vi "I(V) at various fields_K6221-K2182A_PK.vi"() -> ()   [LabVIEW 2016]
uses:
  Labview Drivers/Keithley 622x LV 2009/Keithley 622x.lvlib
panel:
  in  "Numeric Average":i32=1
  out "Iset (A)":dbl=0.000246
  out "data":dbl[](array[numeric])=[-0.004996105, 0.000246, 1.09736792e-07, 0.0004460845203252032]
  out "I vs V":cluster{dbl, "Field Reading":dbl}[](graph)=[{0.0, "Field Reading"=4.05379385e-08}, {2e-06, "Field Reading"=3.64587619e-08}, {4e-06, "Field Reading"=2.9732457e-08}, {6e-06, "Field Reading"=3.98881058e-08}, {8e-06, "Field Reading"=2.30033844e-08}, {1e-05, "Field Reading"=4.97153356e-08}, {1.2e-05, "Field Reading"=4.75621284e-08}, {1.4e-05, "Field Reading"=5.84210222e-08}, {1.6e-05, "Field Reading"=2.26147627e-08}, {1.8e-05, "Field Reading"=5.23454209e-08}, {2e-05, "Field Reading"=6.56079851e-08}, {2.2e-05, "Field Reading"=2.92396798e-08}, {2.4e-05, "Field Reading"=4.16692625e-08}, {2.6e-05, "Field Reading"=4.41799263e-08}, {2.8e-05, "Field Reading"=7.01712601e-08}, {3e-05, "Field Reading"=6.50284783e-08}, {3.2e-05, "Field Reading"=5.58979313e-08}, {3.4e-05, "Field Reading"=5.23483257e-08}, {3.6e-05, "Field Reading"=6.7225832e-08}, {3.8e-05, "Field Reading"=7.54313295e-08}, {4e-05, "Field Reading"=5.53442462e-08}, {4.2e-05, "Field Reading"=4.50714271e-08}, {4.4e-05, "Field Reading"=7.33557968e-08}, {4.6e-05, "Field Reading"=7.29903849e-08}, {4.8e-05, "Field Reading"=6.72053986e-08}, {5e-05, "Field Reading"=7.52270368e-08}, {5.2e-05, "Field Reading"=3.48248368e-08}, {5.4e-05, "Field Reading"=4.25123955e-08}, {5.6e-05, "Field Reading"=3.2735953e-08}, {5.8e-05, "Field Reading"=4.13780643e-08}, {6e-05, "Field Reading"=5.62867915e-08}, {6.2e-05, "Field Reading"=5.58870905e-08}, {6.4e-05, "Field Reading"=6.25632145e-08}, {6.6e-05, "Field Reading"=3.84289851e-08}, {6.8e-05, "Field Reading"=3.14361308e-08}, {7e-05, "Field Reading"=4.48345345e-08}, {7.2e-05, "Field Reading"=4.47084767e-08}, {7.4e-05, "Field Reading"=6.25694969e-08}, {7.6e-05, "Field Reading"=3.79772381e-08}, {7.8e-05, "Field Reading"=5.23238288e-08}, {8e-05, "Field Reading"=5.84721878e-08}, {8.2e-05, "Field Reading"=4.40641633e-08}, {8.4e-05, "Field Reading"=6.65961279e-08}, {8.6e-05, "Field Reading"=4.87730467e-08}, {8.8e-05, "Field Reading"=4.86681064e-08}, {9e-05, "Field Reading"=3.06449251e-08}, {9.2e-05, "Field Reading"=2.04011436e-08}, {9.4e-05, "Field Reading"=3.48937095e-08}, {9.6e-05, "Field Reading"=3.13306358e-08}, {9.8e-05, "Field Reading"=5.74364404e-08}, {0.0001, "Field Reading"=3.84366611e-08}, {0.000102, "Field Reading"=1.84804306e-08}, {0.000104, "Field Reading"=2.93325997e-08}, {0.000106, "Field Reading"=3.33698481e-08}, {0.000108, "Field Reading"=5.53641043e-08}, {0.00011, "Field Reading"=2.20652981e-08}, {0.000112, "Field Reading"=5.83884174e-08}, {0.000114, "Field Reading"=2.35472946e-08}, {0.000116, "Field Reading"=1.33616069e-08}, {0.000118, "Field Reading"=7.07626517e-08}, {0.00012, "Field Reading"=5.73898691e-08}, {0.000122, "Field Reading"=5.68743057e-08}, {0.000124, "Field Reading"=4.35484976e-08}, {0.000126, "Field Reading"=4.87329306e-08}, {0.000128, "Field Reading"=3.3317892e-08}, {0.00013, "Field Reading"=3.10876308e-09}, {0.000132, "Field Reading"=2.26640431e-08}, {0.000134, "Field Reading"=5.22671704e-08}, {0.000136, "Field Reading"=5.63622352e-08}, {0.000138, "Field Reading"=6.76896268e-08}, {0.00014, "Field Reading"=5.1228327e-08}, {0.000142, "Field Reading"=5.78385795e-08}, {0.000144, "Field Reading"=4.15431867e-08}, {0.000146, "Field Reading"=4.45472386e-08}, {0.000148, "Field Reading"=8.49816974e-08}, {0.00015, "Field Reading"=3.95992446e-08}, {0.000152, "Field Reading"=3.29649066e-08}, {0.000154, "Field Reading"=6.66106268e-08}, {0.000156, "Field Reading"=6.30337569e-08}, {0.000158, "Field Reading"=6.35013052e-08}, {0.00016, "Field Reading"=5.83753613e-08}, {0.000162, "Field Reading"=6.14367492e-08}, {0.000164, "Field Reading"=7.53864217e-08}, {0.000166, "Field Reading"=6.10784622e-08}, {0.000168, "Field Reading"=8.04991415e-08}, {0.00017, "Field Reading"=6.00893675e-08}, {0.000172, "Field Reading"=6.36170226e-08}, {0.000174, "Field Reading"=4.4632519e-08}, {0.000176, "Field Reading"=9.8380093e-08}, {0.000178, "Field Reading"=5.74157276e-08}, {0.00018, "Field Reading"=3.59792374e-08}, {0.000182, "Field Reading"=5.59545702e-08}, {0.000184, "Field Reading"=6.66423799e-08}, {0.000186, "Field Reading"=4.972552e-08}, {0.000188, "Field Reading"=4.66398654e-08}, {0.00019, "Field Reading"=5.74303765e-08}, {0.000192, "Field Reading"=8.50804633e-08}, {0.000194, "Field Reading"=6.55690267e-08}, {0.000196, "Field Reading"=5.07497489e-08}, {0.000198, "Field Reading"=3.63764116e-08}, {0.0002, "Field Reading"=3.93241537e-08}, {0.000202, "Field Reading"=4.19967581e-08}, {0.000204, "Field Reading"=5.70078995e-08}, {0.000206, "Field Reading"=7.48360739e-08}, {0.000208, "Field Reading"=8.80933969e-08}, {0.00021, "Field Reading"=7.17906614e-08}, {0.000212, "Field Reading"=7.5446937e-08}, {0.000214, "Field Reading"=4.71850583e-08}, {0.000216, "Field Reading"=7.68570777e-08}, {0.000218, "Field Reading"=3.60011353e-08}, {0.00022, "Field Reading"=6.41115795e-08}, {0.000222, "Field Reading"=1.08732262e-07}, {0.000224, "Field Reading"=6.93958525e-08}, {0.000226, "Field Reading"=8.36841734e-08}, {0.000228, "Field Reading"=7.95819112e-08}, {0.00023, "Field Reading"=1.04093026e-07}, {0.000232, "Field Reading"=9.83568247e-08}, {0.000234, "Field Reading"=1.08221251e-07}, {0.000236, "Field Reading"=8.47085746e-08}, {0.000238, "Field Reading"=9.58289848e-08}, {0.00024, "Field Reading"=8.45457692e-08}, {0.000242, "Field Reading"=1.16904729e-07}, {0.000244, "Field Reading"=1.06152824e-07}, {0.000246, "Field Reading"=1.09736792e-07}]
  in  "wait (ms)":u32=50
  in  "Set Compliance voltage (V)":dbl=10.0 min=0.0 step=0.1 format="%_3f"
  in  "Nanovoltmeter 2182a VISA":refnum<visa-resource-name>="GPIB0::7::INSTR"
  in  "Current source K6221 VISA":refnum<visa-resource-name>="GPIB0::12::INSTR"
  out "Time (s)":dbl=173.162 format="%#_13g"
  in  "Field ramp rate (T/min)":string="0.00001"
  in  "Magnetic field stabilization time (s)":dbl=10.0 format="%#_13g"
  in  "Step 2":dbl[](array[numeric])=[5e-06] min=-3000.0 max=3000.0 format="%.1e"
  in  "To 2":dbl[](array[numeric])=[0.005] min=-3000.0 max=3000.0 format="%.1e"
  in  "From 2":dbl[](array[numeric])=[-0.005] min=-3000.0 max=3000.0 format="%.1e"
  out "Magnetic Field (T)":dbl=-0.004996105 format="%#_13g"
  in  "Magnet IP Address":string="169.254.212.113"
  out "Vmeas (V)":dbl=1.09736792e-07
  in  "Folder":path=path "D:/Pranava/Data/NiTe2/05-02-2022/005/06-04-2022"
  in  "Step":dbl[](array[numeric])=[2e-06, 5e-05, 2e-06, 5e-05] min=-3000.0 max=3000.0 format="%.1e"
  in  "To":dbl[](array[numeric])=[0.0006, 0.0, -0.0006, 0.0] min=-3000.0 max=3000.0 format="%.1e"
  in  "From":dbl[](array[numeric])=[0.0, 0.0006, 0.0, -0.0006] min=-3000.0 max=3000.0 format="%.1e"
  in  "file name":string="018_05-02-2022_NiTe2_005_DevN_DC_IV(H)_map_OOP_Y-axis_baseT(180mK)_I_36-37_V_39-34_5mT_to_5mT"
  out "File path":path=path "D:/Pranava/Data/NiTe2/05-02-2022/005/06-04-2022/018_05-02-2022_NiTe2_005_DevN_DC_IV(H)_map_OOP_Y-axis_baseT(180mK)_I_36-37_V_39-34_5mT_to_5mT.dat"
  # ".dat"
  # "[Must be less than 0.05]"
  # "Configure Magnetic field sweep (T)"
  # "Set Current sweep (A)"
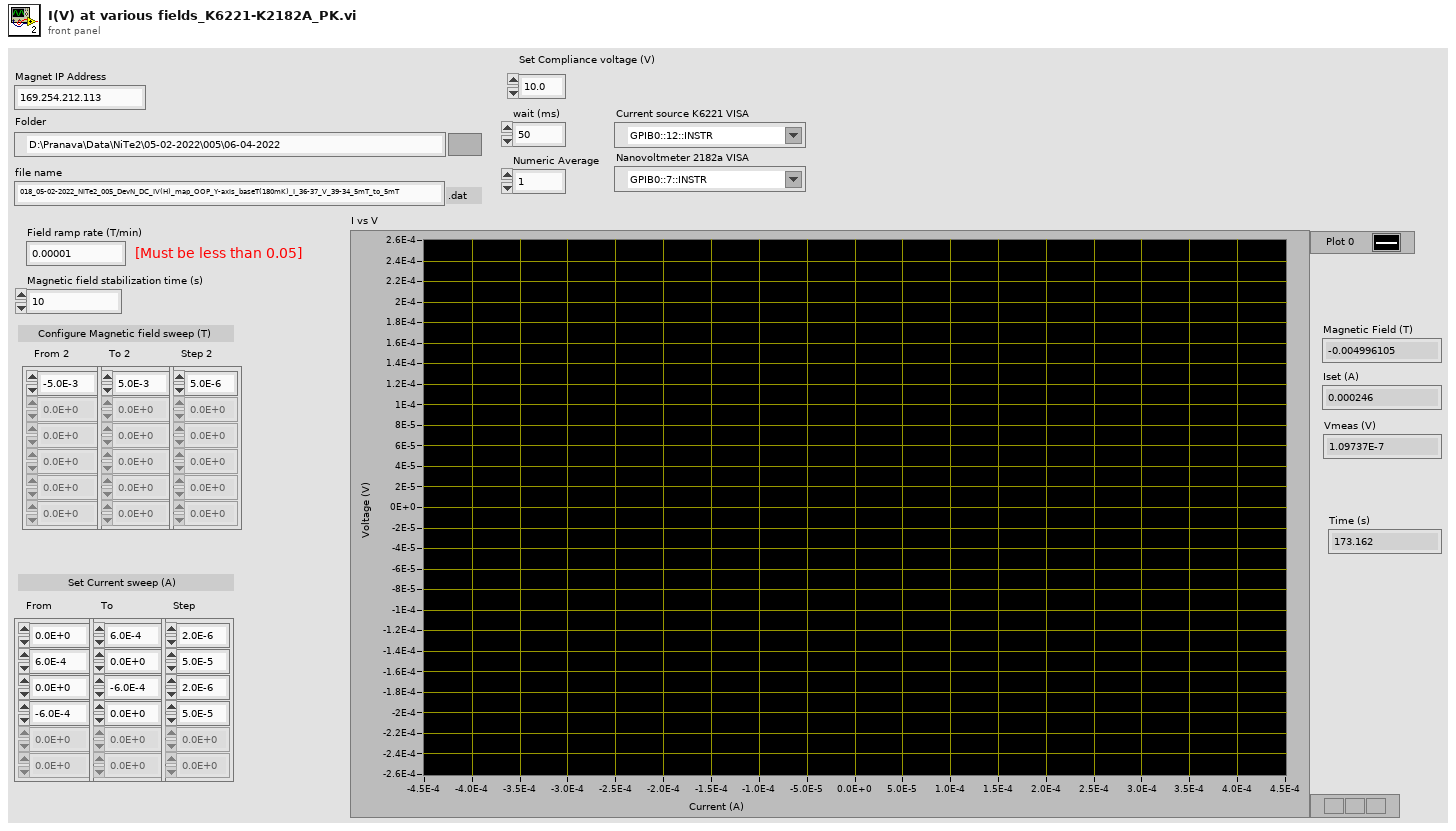
[diagram p1: front panel]
types:
  T1 = enum16{"open", "replace", "create", "open or create", "replace or create", "replace or create with confirmation"}
  T2 = typedef "Keithley 622x.lvlib/KE622x -- Current Level.ctl" = dbl
  T3 = cluster{"Average value":dbl, "Average value":dbl}
  T4 = cluster{"Average value":dbl, "Average value":dbl}[]
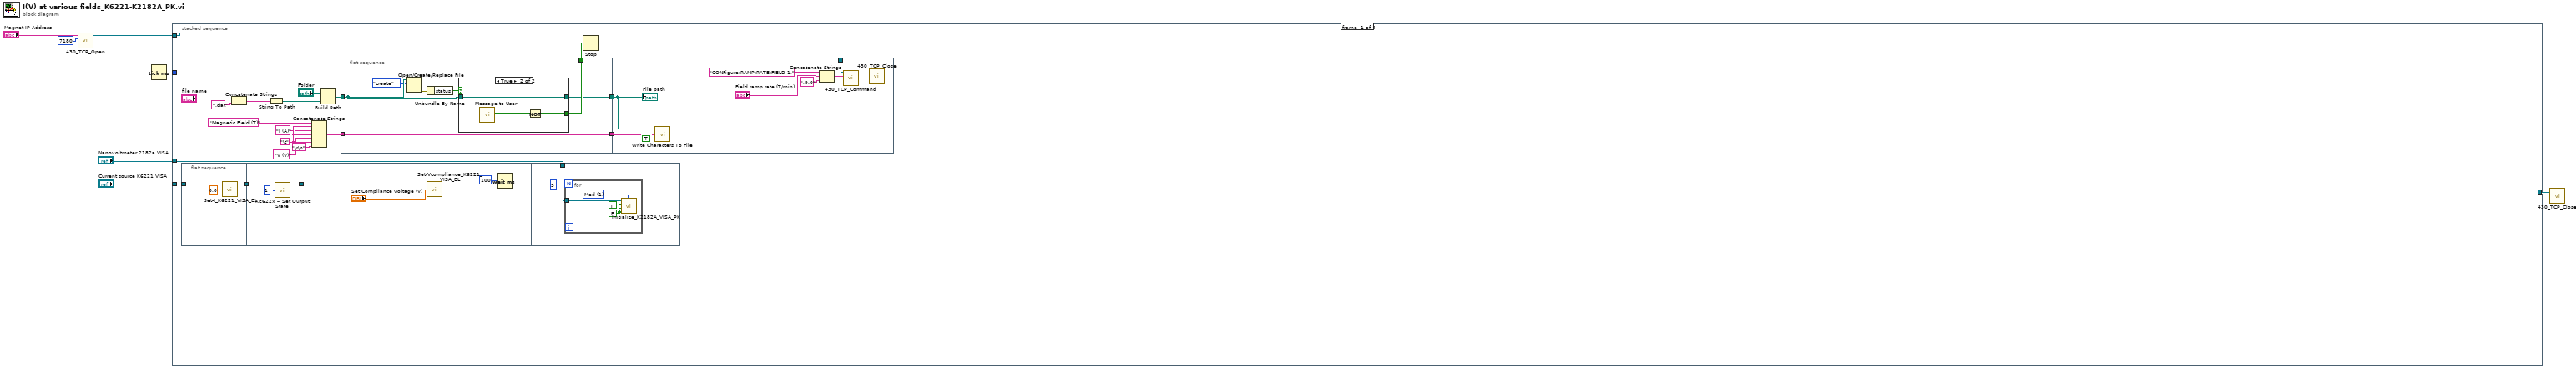
[diagram p0: block diagram]
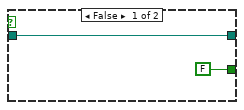
[diagram p2: hidden frame]
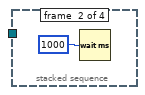
[diagram p3: hidden frame]
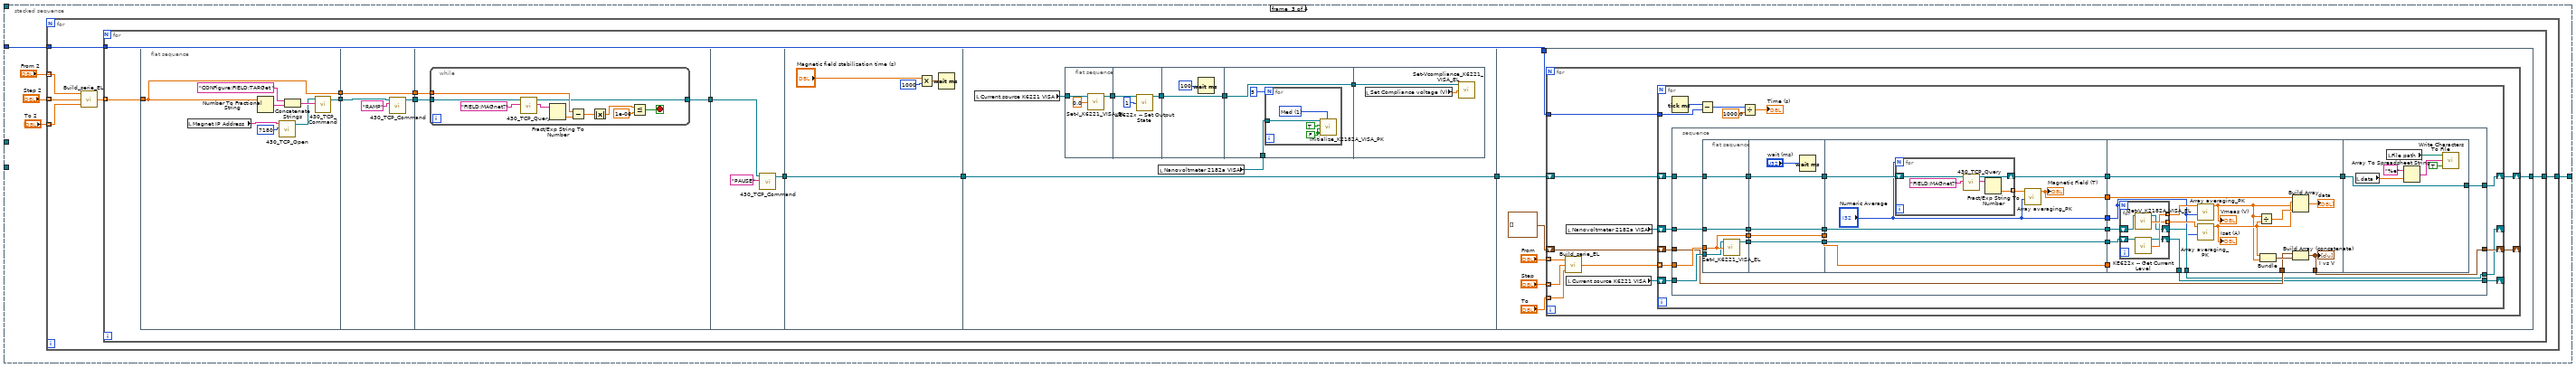
[diagram p4: hidden frame]
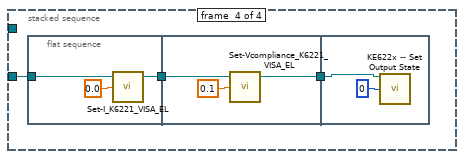
[diagram p5: hidden frame]
diagram:
  n1 = call "430_TCP_Open.vi"("IP Address"="Magnet IP Address", "TCP Port"=7180) -> ("connection ID"=w4:refnum<k5>)  [unwired: 4 in, 2 out]
  n2 = Tick Count (ms)() -> (millisecond timer value=w3:u32)
  n3 = stacked-sequence {
    tunnel: [_ _ w66 _] -> w7
    tunnel: w4 -> [w14 _ _ _]
    tunnel: w3 -> [_ _ w65 _]
    tunnel: "Current source K6221 VISA" -> [w10 _ _ w250]
    tunnel: "Nanovoltmeter 2182a VISA" -> [w9 _ _ _]
    frame #0 {
      w24 = "\t"
      n4 = flat-sequence {
        tunnel: w10 -> [w30]
        tunnel: [w28] -> w11
        tunnel: w11 -> [w33]
        tunnel: [w31] -> w8
        tunnel: w8 -> [w34]
        tunnel: w9 -> [w37]
        frame #0 {
          n5 = call "Set-I_K6221_VISA_EL.vi"("Set I (A)"=0.0, "K6221 VISA"=w30) -> ("K6221 VISA out"=w28:refnum<visa-resource-name>)  [unwired: 2 in, 1 out]
        }
        frame #1 {
          n6 = call "KE622x -- Set Output State.vi"("Resource In"=w33, "Output State"=1) -> ("Resource Out (dupl)"=w31:refnum<visa-resource-name>)  [unwired: 12 in, 1 out]
        }
        frame #2 {
          n7 = call "Set-Vcompliance_K6221_VISA_EL.vi"("Set Compliance voltage (V)"="Set Compliance voltage (V)", "K6221 VISA"=w34) -> ()  [unwired: 2 in, 2 out]
        }
        frame #3 {
          n8 = Wait (ms)(milliseconds to wait=100) -> ()  [unwired: 1 out]
        }
        frame #4 {
          n9 = for {
            N: 5 ("Numeric") -> [_]
            tunnel: w37 -> [w39]
            w41 = u16 1 items=["Slow", "Med", "Fast"] ("Rate (NPLC)")
            w42 = FALSE ("Auto range?")
            n10 = call "Initialize_K2182A_VISA_PK.vi"("VISA address"=w39, "Auto range?"=TRUE, "Analog LPass\nFilter?"=w42, "DC\nFilter?"=w42, "Rate (NPLC)"=w41) -> ()  [unwired: 2 in]
          }
        }
      }
      n11 = Concatenate Strings("file name", ".dat" ("string")) -> (w22:string)
      n12 = String To Path(string=w22) -> (path=w16:path)
      n13 = Concatenate Strings("Magnetic Field (T)", w24, "I (A)" ("string"), w24, "V (V)" ("string"), w24, "\r\n") -> (w23:string)
      n14 = Build Path(base path="Folder", name or relative path=w16) -> (appended path=w15:path)
      n15 = flat-sequence {
        tunnel: w15 -> [w46]
        tunnel: w23 -> [w49]
        tunnel: [w49] -> w27
        tunnel: [w48] -> w20
        tunnel: [w47] -> w26
        tunnel: w27 -> [w56]
        tunnel: w26 -> [w55]
        tunnel: w14 -> [w58]
        frame #0 {
          n16 = Open/Create/Replace File(file path (use dialog)=w46, operation (0:open)=T1."create") -> (error out=w45:errorcluster)  [unwired: 4 in, 2 out]
          n17 = Unbundle By Name(w45) -> ("status"=w43:bool)
          n18 = case shown="True" w43 {
            tunnel: [FALSE ("Yes") w53] -> w48
            tunnel: [w50 w52] -> w47
            tunnel: w46 -> [w50 w52]
            frame False {
            }
            frame True {
              n19 = call "Message to User"() -> ("Yes"=w54:bool)  [unwired: 10 in, 1 out]
              n20 = Not(x=w54) -> (.not. x?=w53:bool)
            }
          }
        }
        frame #1 {
          n21 = call <vilib>:"Write Characters To File.vi"("append to file? (new file:F)"=TRUE, "character string"=w56, "file path (dialog if empty)"=w55) -> ()  [unwired: 2 in, 1 out]
          "File path" <- w55
        }
        frame #2 {
          n22 = Concatenate Strings("CONFigure:RAMP:RATE:FIELD 1," ("String"), "Field ramp rate (T/min)", ",9.0") -> (w59:string)
          n23 = call "430_TCP_Command.vi"("Command"=w59, "connection ID"=w58) -> ("connection ID out"=w63:refnum<k5>)  [unwired: 2 in, 2 out]
          n24 = call "430_TCP_Close.vi"("connection ID"=w63) -> ()  [unwired: 1 in, 2 out]
        }
      }
      n25 = Stop(stop? (T)=w20) -> ()
    }
    frame #1 {
      n26 = Wait (ms)(milliseconds to wait=u32 1000) -> ()  [unwired: 1 out]
    }
    frame #2 {
      n27 = for {
        tunnel: "From 2" -> [w75] mode=indexing
        tunnel: "To 2" -> [w73] mode=indexing
        tunnel: "Step 2" -> [w74] mode=indexing
        tunnel: [w71] -> w66
        tunnel: w65 -> [w70]
        n28 = call "Build_serie_EL.vi"("end value"=w73, "increment"=w74, "start value"=w75) -> ("output array"=w72:dbl[])
        n29 = for {
          tunnel: w72 -> [w86] mode=indexing
          tunnel: [w83] -> w71
          tunnel: w70 -> [w80]
          n30 = flat-sequence {
            tunnel: w86 -> [w90]
            tunnel: [w91] -> w82
            tunnel: [w90] -> w81
            tunnel: [w96] -> w85
            tunnel: [w95] -> w84
            tunnel: w81 -> [w95]
            tunnel: w82 -> [w98]
            tunnel: w85 -> [w101]
            tunnel: w84 -> [w100]
            tunnel: [w99] -> w77
            tunnel: w77 -> [w114]
            tunnel: [w113] -> w76
            tunnel: [w115] -> w79
            tunnel: w76 -> [w115]
            tunnel: w79 -> [w125]
            tunnel: [w125] -> w78
            tunnel: w78 -> [w146]
            tunnel: [w145] -> w83
            tunnel: w80 -> [w144]
            frame #0 {
              n31 = local read "Magnet IP Address"() -> (w88:string)
              n32 = Number To Fractional String(number=w90) -> (F-format string=w92:string)  [unwired: 3 in]
              n33 = call "430_TCP_Open.vi"("IP Address"=w88, "TCP Port"=7180) -> ("connection ID"=w87:refnum<k5>)  [unwired: 4 in, 2 out]
              n34 = Concatenate Strings("CONFigure:FIELD:TARGet " ("String"), w92) -> (w94:string)
              n35 = call "430_TCP_Command.vi"("Command"=w94, "connection ID"=w87) -> ("connection ID out"=w91:refnum<k5>)  [unwired: 2 in, 2 out]
            }
            frame #1 {
              n36 = call "430_TCP_Command.vi"("Command"="RAMP", "connection ID"=w98) -> ("connection ID out"=w96:refnum<k5>)  [unwired: 2 in, 2 out]
            }
            frame #2 {
              n37 = while {
                tunnel: w101 -> [w111]
                tunnel: w100 -> [w106]
                tunnel: [w102] -> w99
                stop <- w104 stop-if-true
                n38 = call "430_TCP_Query.vi"("Command"="FIELD:MAGnet?" ("String"), "connection ID"=w111) -> ("Response"=w110:string, "connection ID out"=w102:refnum<k5>)  [unwired: 5 in, 3 out]
                n39 = Fract/Exp String To Number(string=w110) -> (number=w107:dbl)  [unwired: 3 in, 1 out]
                n40 = Subtract(x=w106, y=w107) -> (x-y=w109:dbl)
                n41 = Absolute Value(x=w109) -> (abs(x)=w108:dbl)
                n42 = Less Or Equal?(x=w108, y=1e-06) -> (x <= y?=w104:bool)
              }
            }
            frame #3 {
              n43 = call "430_TCP_Command.vi"("Command"="PAUSE", "connection ID"=w114) -> ("connection ID out"=w113:refnum<k5>)  [unwired: 2 in, 2 out]
            }
            frame #4 {
              n44 = Multiply(x="Magnetic field stabilization time (s)", y=1000) -> (x*y=w117:dbl)
              n45 = Wait (ms)(milliseconds to wait=w117) -> ()  [unwired: 1 out]
            }
            frame #5 {
              n46 = local read "Current source K6221 VISA"() -> (w120:refnum<visa-resource-name>)
              n47 = flat-sequence {
                tunnel: w120 -> [w128]
                tunnel: [w126] -> w124
                tunnel: w124 -> [w131]
                tunnel: [w129] -> w123
                tunnel: w123 -> [w132]
                tunnel: [w132] -> w122
                tunnel: w122 -> [w135]
                tunnel: [w135] -> w121
                tunnel: w119 -> [w134]
                tunnel: w121 -> [w141]
                frame #0 {
                  n48 = call "Set-I_K6221_VISA_EL.vi"("Set I (A)"=0.0, "K6221 VISA"=w128) -> ("K6221 VISA out"=w126:refnum<visa-resource-name>)  [unwired: 2 in, 1 out]
                }
                frame #1 {
                  n49 = call "KE622x -- Set Output State.vi"("Resource In"=w131, "Output State"=1) -> ("Resource Out (dupl)"=w129:refnum<visa-resource-name>)  [unwired: 12 in, 1 out]
                }
                frame #2 {
                  n50 = Wait (ms)(milliseconds to wait=100) -> ()  [unwired: 1 out]
                }
                frame #3 {
                  n51 = for {
                    N: 5 ("Numeric") -> [_]
                    tunnel: w134 -> [w137]
                    w139 = u16 1 items=["Slow", "Med", "Fast"] ("Rate (NPLC)")
                    w140 = FALSE ("Auto range?")
                    n52 = call "Initialize_K2182A_VISA_PK.vi"("VISA address"=w137, "Auto range?"=TRUE, "Analog LPass\nFilter?"=w140, "DC\nFilter?"=w140, "Rate (NPLC)"=w139) -> ()  [unwired: 2 in]
                  }
                }
                frame #4 {
                  n53 = local read "Set Compliance voltage (V)"() -> (w142:dbl)
                  n54 = call "Set-Vcompliance_K6221_VISA_EL.vi"("Set Compliance voltage (V)"=w142, "K6221 VISA"=w141) -> ()  [unwired: 2 in, 2 out]
                }
              }
              n55 = local read "Nanovoltmeter 2182a VISA"() -> (w119:refnum<visa-resource-name>)
            }
            frame #6 {
              n56 = for {
                tunnel: "From" -> [w158] mode=indexing
                tunnel: "To" -> [w157] mode=indexing
                tunnel: "Step" -> [w156] mode=indexing
                shift-right: [w160] -> _
                shift-left: cluster{dbl, "Field Reading":dbl}[] [] -> [w150]
                shift-right: [w154] -> w145
                shift-left: w146 -> [w155]
                tunnel: w144 -> [w153]
                n57 = call "Build_serie_EL.vi"("end value"=w157, "increment"=w156, "start value"=w158) -> ("output array"=w159:dbl[])
                n58 = local read "Nanovoltmeter 2182a VISA"() -> (w151:refnum<visa-resource-name>)
                n59 = local read "Current source K6221 VISA"() -> (w152:refnum<visa-resource-name>)
                n60 = for {
                  tunnel: w159 -> [w174] mode=indexing
                  shift-right: [w172] -> w160
                  shift-left: w150 -> [w173]
                  shift-right: [w161] -> _
                  shift-left: w152 -> [w171]
                  shift-right: [w162] -> _
                  shift-left: w151 -> [w170]
                  shift-right: [w169] -> w154
                  shift-left: w155 -> [w168]
                  tunnel: w153 -> [w164]
                  n61 = Tick Count (ms)() -> (millisecond timer value=w165:u32)
                  n62 = stacked-sequence {
                    tunnel: w174 -> [w198]
                    tunnel: w173 -> [w186]
                    tunnel: [w185] -> w172
                    tunnel: w171 -> [w197]
                    tunnel: w170 -> [w196]
                    tunnel: [w192] -> w169
                    tunnel: w168 -> [w191]
                    tunnel: [w177] -> w162
                    tunnel: [w176] -> w161
                    frame #0 {
                      n63 = flat-sequence {
                        tunnel: [w202] -> w190
                        tunnel: [w203] -> w188
                        tunnel: w191 -> [w203]
                        tunnel: w196 -> [w199]
                        tunnel: w197 -> [w201]
                        tunnel: w198 -> [w202]
                        tunnel: [w200] -> w182
                        tunnel: [w199] -> w181
                        tunnel: w190 -> [w208]
                        tunnel: [w208] -> w189
                        tunnel: w188 -> [w207]
                        tunnel: [w207] -> w187
                        tunnel: [w205] -> w183
                        tunnel: w182 -> [w205]
                        tunnel: w181 -> [w204]
                        tunnel: [w204] -> w180
                        tunnel: w189 -> [w216]
                        tunnel: [w216] -> w195
                        tunnel: [w210] -> w194
                        tunnel: [w215] -> w193
                        tunnel: w187 -> [w214]
                        tunnel: [w213] -> w184
                        tunnel: w183 -> [w213]
                        tunnel: w180 -> [w212]
                        tunnel: [w212] -> w179
                        tunnel: ["Numeric Average"] -> w175
                        tunnel: w193 -> [w237]
                        tunnel: w194 -> [w227]
                        tunnel: w195 -> [_]
                        tunnel: w186 -> [w231]
                        tunnel: [w230] -> w185
                        tunnel: w184 -> [w229]
                        tunnel: w179 -> [w228]
                        tunnel: [w237] -> w178
                        tunnel: [w224] -> w177
                        tunnel: [w223] -> w176
                        tunnel: w175 -> [w222]
                        tunnel: [w249] -> w192
                        tunnel: w178 -> [w249]
                        frame #0 {
                          n64 = call "Set-I_K6221_VISA_EL.vi"("Set I (A)"=w202, "K6221 VISA"=w201) -> ("K6221 VISA out"=w200:refnum<visa-resource-name>)  [unwired: 2 in, 1 out]
                        }
                        frame #1 {
                          n65 = Wait (ms)(milliseconds to wait="wait (ms)") -> ()  [unwired: 1 out]
                        }
                        frame #2 {
                          n66 = for {
                            N: "Numeric Average" -> [_]
                            tunnel: [w219] -> w211 mode=indexing
                            shift-right: [w218] -> w215
                            shift-left: w214 -> [w217]
                            n67 = call "430_TCP_Query.vi"("Command"="FIELD:MAGnet?" ("String"), "connection ID"=w217) -> ("Response"=w221:string, "connection ID out"=w218:refnum<k5>)  [unwired: 5 in, 3 out]
                            n68 = Fract/Exp String To Number(string=w221) -> (number=w219:dbl)  [unwired: 3 in, 1 out]
                          }
                          n69 = call "Array averaging_PK.vi"("Number averaging"="Numeric Average", "numeric array"=w211) -> ("Average value"=w210:dbl)  [unwired: 9 in]
                          "Magnetic Field (T)" <- w210
                        }
                        frame #3 {
                          n70 = for {
                            N: w222 -> [_]
                            tunnel: [w243] -> w234 mode=indexing
                            tunnel: [w242] -> w233 mode=indexing
                            shift-right: [w240] -> w223
                            shift-left: w229 -> [w241]
                            shift-right: [w238] -> w224
                            shift-left: w228 -> [w239]
                            n71 = call "Get-V_K2182A_VISA_EL.vi"("VISA K2182A"=w239) -> ("V (V)"=w243:dbl, "VISA K2182A"=w238:refnum<visa-resource-name>)  [unwired: 2 in, 1 out]
                            n72 = call "KE622x -- Get Current Level.vi"("Resource In"=w241) -> ("Resource Out (dupl)"=w240:refnum<visa-resource-name>, "Current Level (A)"=w242:T2)  [unwired: 12 in, 1 out]
                          }
                          n73 = call "Array averaging_PK.vi"("Number averaging"=w222, "numeric array"=w234) -> ("Average value"=w225:dbl)  [unwired: 9 in]
                          "Vmeas (V)" <- w225
                          n74 = call "Array averaging_PK.vi"("Number averaging"=w222, "numeric array"=w233) -> ("Average value"=w226:dbl)  [unwired: 9 in]
                          "Iset (A)" <- w226
                          n75 = Divide(x=w225, y=w226) -> (x/y=w232:dbl)
                          n76 = Bundle("Average value"=w226, "Average value"=w225) -> (w235:T3)  [unwired: 1 in]
                          n77 = Build Array(w227, w226, w225, w232) -> (→"data":dbl[])
                          n78 = Build Array (concatenate)(w231, w235) -> (w230:T4)
                          "I vs V" <- w230
                        }
                        frame #4 {
                          n79 = local read "data"() -> (w244:dbl[])
                          n80 = local read "File path"() -> (w246:path)
                          n81 = Array To Spreadsheet String(array=w244, 3:"%e" ("format string")) -> (spreadsheet string=w247:string)  [unwired: 1 in]
                          n82 = call <vilib>:"Write Characters To File.vi"("append to file? (new file:F)"=TRUE, "character string"=w247, "file path (dialog if empty)"=w246) -> ()  [unwired: 2 in, 1 out]
                        }
                      }
                    }
                  }
                  n83 = Subtract(x=w165, y=w164) -> (x-y=w167:u32)
                  n84 = Divide(x=w167, y=1000.0) -> (x/y=→"Time (s)":dbl)
                }
              }
            }
          }
        }
      }
    }
    frame #3 {
      n85 = flat-sequence {
        tunnel: w250 -> [w255]
        tunnel: [w253] -> w252
        tunnel: w252 -> [w257]
        tunnel: [w256] -> w251
        tunnel: w251 -> [w260]
        frame #0 {
          n86 = call "Set-I_K6221_VISA_EL.vi"("Set I (A)"=0.0, "K6221 VISA"=w255) -> ("K6221 VISA out"=w253:refnum<visa-resource-name>)  [unwired: 2 in, 1 out]
        }
        frame #1 {
          n87 = call "Set-Vcompliance_K6221_VISA_EL.vi"("Set Compliance voltage (V)"=0.1, "K6221 VISA"=w257) -> ("K6221 VISA out"=w256:refnum<visa-resource-name>)  [unwired: 2 in, 1 out]
        }
        frame #2 {
          n88 = call "KE622x -- Set Output State.vi"("Resource In"=w260, "Output State"=0) -> ()  [unwired: 12 in, 2 out]
        }
      }
    }
  }
  n89 = call "430_TCP_Close.vi"("connection ID"=w7) -> ()  [unwired: 1 in, 2 out]
